vi "LogError.vi"(8 "error in (no error)":errorcluster, 11 "TCP_serverGUI in":refnum<class "TCP_serverGUI.lvclass">) -> (0 "error out":errorcluster, 3 "TCP_serverGUI out":refnum<class "TCP_serverGUI.lvclass">)   [LabVIEW 2023, in "TCP_serverGUI.lvlib" / "TCP_serverGUI.lvclass"]
uses:
  TCP_serverGUI.lvclass
  TCP_serverGUI.lvclass/TCP_serverGUI.ctl
  SimpleErrorLogger/SimpleErrorLogger Messages/LogError Msg/LogError Msg.lvclass
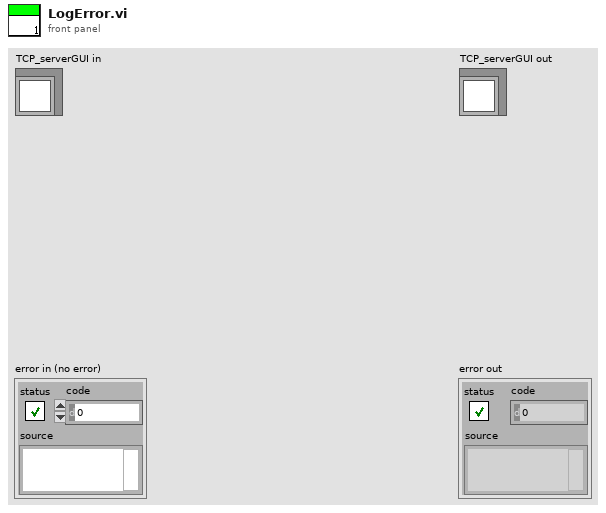
[diagram p1: front panel]
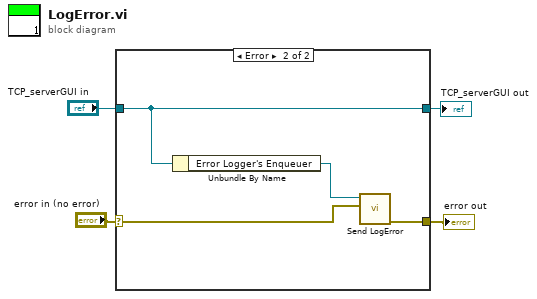
[diagram p0: block diagram]
diagram:
  n1 = case shown="Error" "error in (no error)" {
    selector: "error in (no error)" -> [w5 w8]
    tunnel: [w5 w7] -> w3
    tunnel: [w6 w10] -> w1
    tunnel: "TCP_serverGUI in" -> [w6 w10]
    frame No Error {
    }
    frame Error {
      n2 = Unbundle By Name(w10) -> ("Error Logger's Enqueuer"=w9:refnum<class "Message Enqueuer.lvclass">)
      n3 = call "Send LogError.vi"("error"=w8, "Message Enqueuer"=w9) -> ("error out"=w7:errorcluster)  [unwired: 8 in, 1 out]
    }
  }
  "error out" <- w3
  "TCP_serverGUI out" <- w1
